vi "Run.vi"(8 "error in (no error)":errorcluster, 11 "RealBattery in":refnum<class "RealBattery.lvclass">) -> (0 "error out":errorcluster, 3 "RealBattery out":refnum<class "RealBattery.lvclass">)   [LabVIEW 2013, in "RealBattery.lvclass"]
uses:
  RealBattery.lvclass
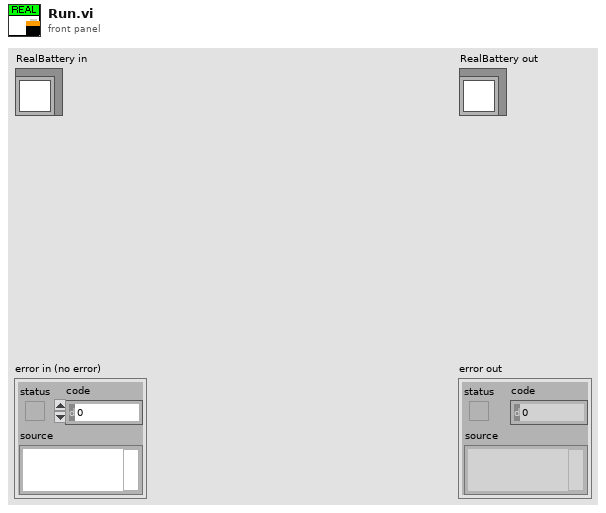
[diagram p1: front panel]
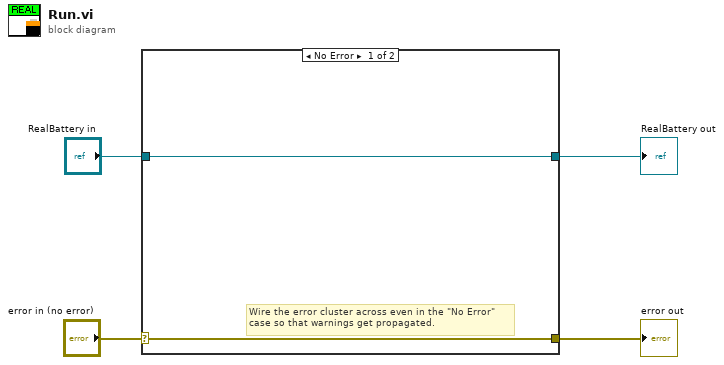
[diagram p0: block diagram]
diagram:
  n1 = case shown="No Error" "error in (no error)" {
    selector: "error in (no error)" -> [w6 w8]
    tunnel: [w6 w8] -> w1
    tunnel: [w5 w7] -> w2
    tunnel: "RealBattery in" -> [w5 w7]
    frame No Error {
      # "Wire the error cluster across even in the \"No Error\"\ncase so that warnings get propagated."
    }
    frame Error {
    }
  }
  "error out" <- w1
  "RealBattery out" <- w2
